vi "MultiBiasScan.vi"() -> ()   [LabVIEW 2014]
uses:
  <userlib>/Nanonis Prog Interface V5/Nanonis Prog Interface.lvlib
panel:
  out "Progress":u8(slide) scale=0.0..1.0
  out "Current":dbl format="%#_6p"
  out "Bias":dbl format="%#_6p"
  in  "Scans":i32[](listbox)
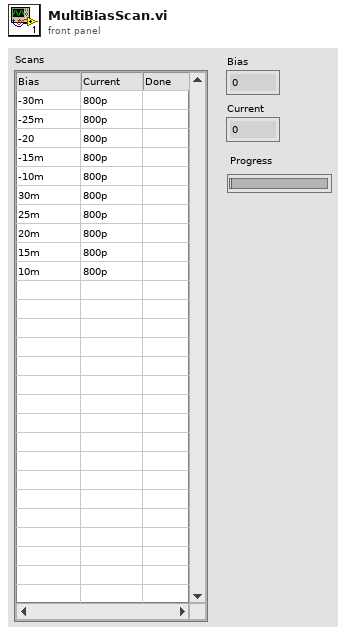
[diagram p1: front panel]
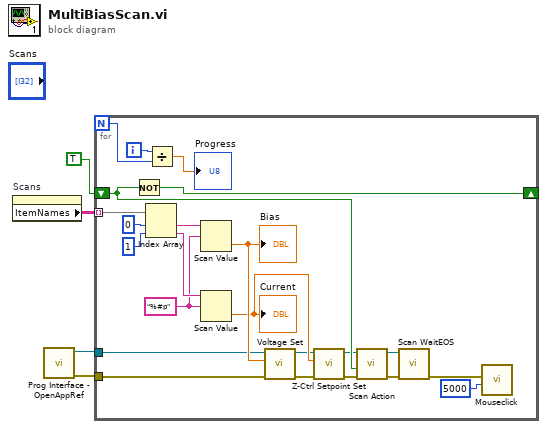
[diagram p0: block diagram]
diagram:
  n1 = property on="Scans" class="MCListbox (strict)"() -> ("ItemNames"=w3:string[][])  [unwired: 2 in, 2 out]
  n2 = call <userlib>:"Prog Interface - OpenAppRef.vi"() -> ("Error out"=w1:errorcluster, "Application reference"=w2:refnum<vi>)  [unwired: 6 in]
  n3 = for {
    N -> [w10]
    tunnel: w3 -> [w27] mode=indexing
    shift-right: [w18] -> _
    shift-left: TRUE ("Direction: up/down (T=up)") -> [w19]
    tunnel: w2 -> [w16]
    tunnel: w1 -> [w15]
    i -> [w12]
    w22 = "%#p" ("format string")
    n4 = Not(x=w19) -> (.not. x?=w18:bool)
    n5 = Index Array(array=w27, index #1=0 ("index"), index #2=1 ("index")) -> (element #1=w24:string, element #2=w23:string)
    n6 = Divide(x=w12, y=w10) -> (x/y=→"Progress":dbl)
    n7 = Scan Value(string=w24, format string=w22) -> (value=w17:dbl)  [unwired: 1 in, 1 out]
    "Bias" <- w17
    n8 = Scan Value(string=w23, format string=w22) -> (value=w7:dbl)  [unwired: 1 in, 1 out]
    "Current" <- w7
    n9 = call <userlib>:"Voltage Set.vi"("Error in (no error)"=w15, "Bias (V)"=w17, "Application ref in"=w16) -> ("Error out"=w9:errorcluster, "Application ref out"=w6:refnum<vi>)  [unwired: 7 in]
    n10 = call <userlib>:"Z-Ctrl Setpoint Set.vi"("error in (no error)"=w9, "Z Controller setpoint"=w7, "Application ref in"=w6) -> ("error out"=w8:errorcluster, "Application ref out"=w5:refnum<vi>)  [unwired: 7 in]
    n11 = call <userlib>:"Scan Action.vi"("error in (no error)"=w8, "Direction: up/down (T=up)"=w19, "Application ref in"=w5) -> ("error out"=w21:errorcluster, "Application ref out"=w20:refnum<vi>)  [unwired: 6 in]
    n12 = call <userlib>:"Scan WaitEOS.vi"("error in (no error)"=w21, "Application ref in"=w20) -> ("error out"=w14:errorcluster)  [unwired: 5 in, 3 out]
    n13 = call "Mouseclick.vi"("nMilliseconds"=5000, "error in (no error)"=w14) -> ()  [unwired: 9 in, 1 out]
  }
